vi "task_1.vi"() -> ()   [LabVIEW 2020]
panel:
  out "Score":i32
  in  "Player1":string
  in  "Blue":bool
  out "Blue LED":bool
  in  "Red":bool
  out "Red LED":bool
  in  "Green":bool
  out "Green LED":bool
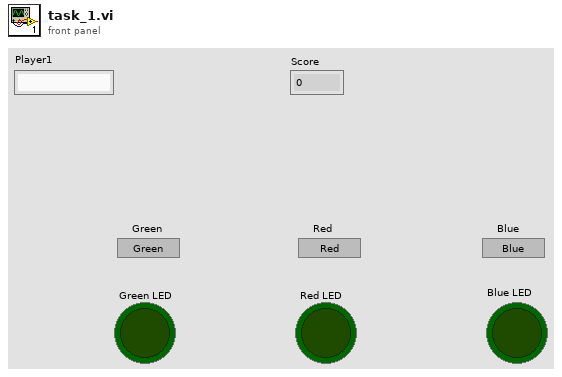
[diagram p1: front panel]
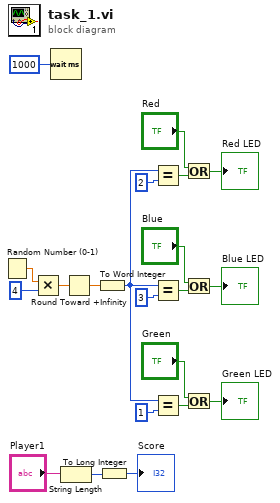
[diagram p0: block diagram]
diagram:
  n1 = Random Number (0-1)() -> (number: 0 to 1=w21:dbl)
  n2 = Multiply(x=w21, y=4) -> (x*y=w20:dbl)
  n3 = Wait (ms)(milliseconds to wait=1000) -> ()  [unwired: 1 out]
  n4 = String Length(string="Player1") -> (length=w3:i32)
  n5 = Round Toward +Infinity(x=w20) -> (ceil(x): smallest int >= x=w18:dbl)
  n6 = To Word Integer(number=w18) -> (16bit integer=w8:i16)
  n7 = To Long Integer(number=w3) -> (32bit integer=→"Score":i32)
  n8 = Equal?(x=w8, y=2) -> (x = y?=w12:bool)
  n9 = Equal?(x=w8, y=3) -> (x = y?=w14:bool)
  n10 = Equal?(x=w8, y=1) -> (x = y?=w17:bool)
  n11 = Or(x="Red", y=w12) -> (x .or. y?=→"Red LED":bool)
  n12 = Or(x="Blue", y=w14) -> (x .or. y?=→"Blue LED":bool)
  n13 = Or(x="Green", y=w17) -> (x .or. y?=→"Green LED":bool)
